vi "main.vi"() -> ()   [LabVIEW 2020]
uses:
  C:/Users/simod/Desktop/Meta/PCanCommunication/Hardware.Can.Peak/bin/Debug/Hardware.Can.Peak.dll
  Hardware.Can.Peak/bin/Debug/Hardware.Can.Peak.dll
  C:/Users/simod/Desktop/Meta/PCanCommunication/Hardware.Can/bin/Debug/Hardware.Can.dll
  Hardware.Can/bin/Debug/Hardware.Can.dll
panel:
  out "Resistance chart [Ohm]":u32(graph)
  out "Actual resistance subarray reversed":u8[](array[numeric])
  out "Actual resistance subarray":u8[](array[numeric])
  out "Actual resistance value [Ohm]":u32
  in  "stop":bool
  out "Actual resistance as hex array":u8[](array[numeric]) format="%x"
  # "Press this button to stop the application in order to release  the CAN resource!"
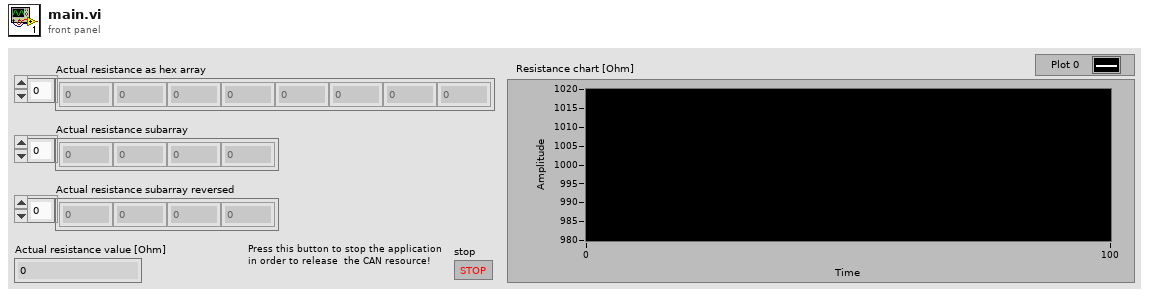
[diagram p1: front panel]
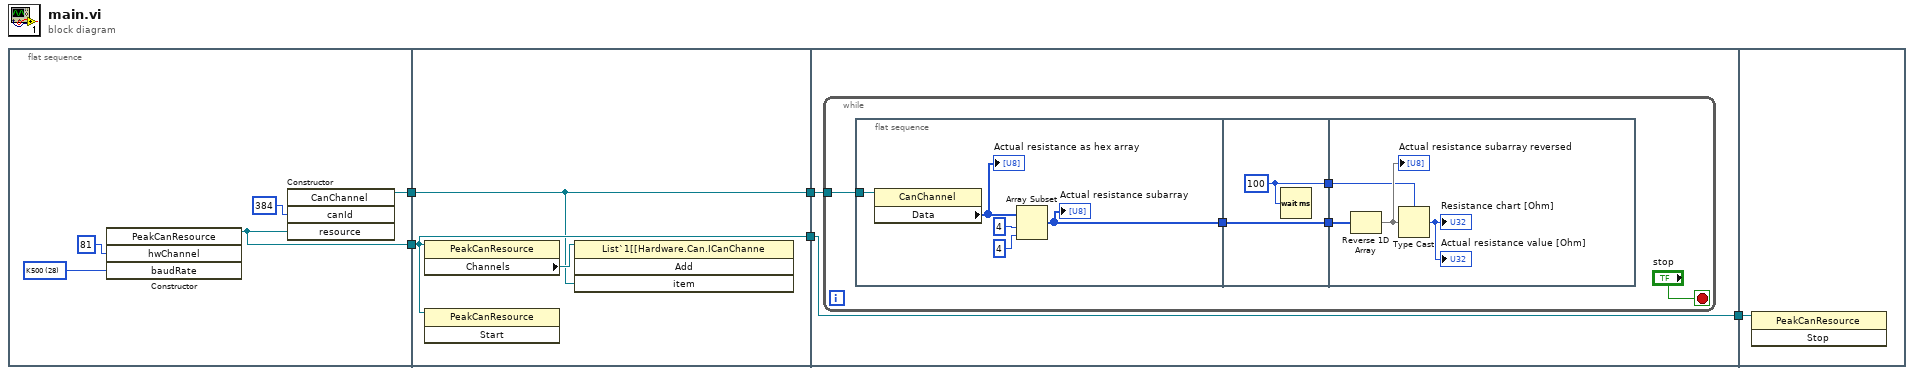
[diagram p0: block diagram]
diagram:
  n1 = flat-sequence {
    tunnel: [w6] -> w5
    tunnel: [w7] -> w4
    tunnel: w5 -> [w12]
    tunnel: w4 -> [w11]
    tunnel: [w11] -> w3
    tunnel: [w12] -> w2
    tunnel: w3 -> [w14]
    tunnel: w2 -> [w15]
    tunnel: [w15] -> w1
    tunnel: w1 -> [w32]
    frame #0 {
      w9 = u16 28 items=["K1000"=20, "K800"=22, "K500"=28, "K250"=284, "K125"=796, "K47"=5140, "K100"=17199, "K50"=18223, "K20"=21295, "K10"=26415, "K5"=32639, "K83"=34091, "K33"=35631, "K95"=49998] ("baudRate")
      n2 = constructor class="PeakCanResource"("hwChannel"=u16 81, "baudRate"=w9) -> (reference out=w6:refnum<k24>)  [unwired: 3 in, 4 out]
      n3 = constructor class="CanChannel"("canId"=384, "resource"=w6) -> (reference out=w7:refnum<k24>)  [unwired: 3 in, 4 out]
    }
    frame #1 {
      n4 = property class="PeakCanResource"(reference=w12) -> ("Channels"=w13:refnum<k24>)  [unwired: 1 in, 2 out]
      n5 = invoke class="PeakCanResource" method="Start"(reference=w12) -> ()  [unwired: 2 in, 3 out]
      n6 = invoke class="List`1[[Hardware.Can.ICanChanne" method="Add"(reference=w13, "item"=w11) -> ()  [unwired: 2 in, 4 out]
    }
    frame #2 {
      n7 = while {
        tunnel: w14 -> [w19]
        stop <- "stop" stop-if-true
        n8 = flat-sequence {
          tunnel: w19 -> [w25]
          tunnel: [w21] -> w18
          tunnel: w18 -> [w27]
          tunnel: [w27] -> w17
          tunnel: [w26] -> w16
          tunnel: w17 -> [w31]
          tunnel: w16 -> [w28]
          frame #0 {
            n9 = property class="CanChannel"(reference=w25) -> ("Data"=w24:u8[])  [unwired: 1 in, 2 out]
            "Actual resistance as hex array" <- w24
            n10 = Array Subset(array=w24, index=4, length=4) -> (w21:u8[])
            "Actual resistance subarray" <- w21
          }
          frame #1 {
            w26 = u32 100 ("milliseconds to wait")
            n11 = Wait (ms)(milliseconds to wait=w26) -> ()  [unwired: 1 out]
          }
          frame #2 {
            n12 = Reverse 1D Array(array=w31) -> (reversed array=w30:u8[])
            "Actual resistance subarray reversed" <- w30
            n13 = Type Cast(type=w28, x=w30) -> (*(type *) &x=→"Actual resistance value [Ohm]" →"Resistance chart [Ohm]":u32)
          }
        }
      }
    }
    frame #3 {
      n14 = invoke class="PeakCanResource" method="Stop"(reference=w32) -> ()  [unwired: 2 in, 3 out]
    }
  }
